vi "(TestVI)RTP Play Test.vi"(5 "RTP Event":refnum<user-event>, 6 "Sampling Rate":u32=8000, 7 "Stop Queue":refnum<queue>, 8 "error in (no error)":errorcluster caption="에러 입력(에러 없음)", 11 "RTP Data":i8[](array[numeric])) -> (0 "error out":errorcluster caption="에러 출력")   [LabVIEW 2020]
uses:
  SubVIs/Serial/Controls/(Ctrl)Serial_Write Read Option.ctl
  f3c870e7-e4f9-4653-aed4-0900bdacb438.vi
  a87611fc-5de5-47b6-9d4c-4620345c1726.vi
  Variables/(Var)System Variables.vi
  SubVIs/Serial/Instance VIs/(SubVI)Serial_Write.vi
  SubVIs/Serial/Instance VIs/(SubVI)Serial_Write-Read.vi
panel:
  out "iteration":i32
  out "Read Array":u8[][](array[numeric])
  out "Current Read":u8[](array[numeric])
  out "time":u32
  out "End Read":u8[](array[numeric])
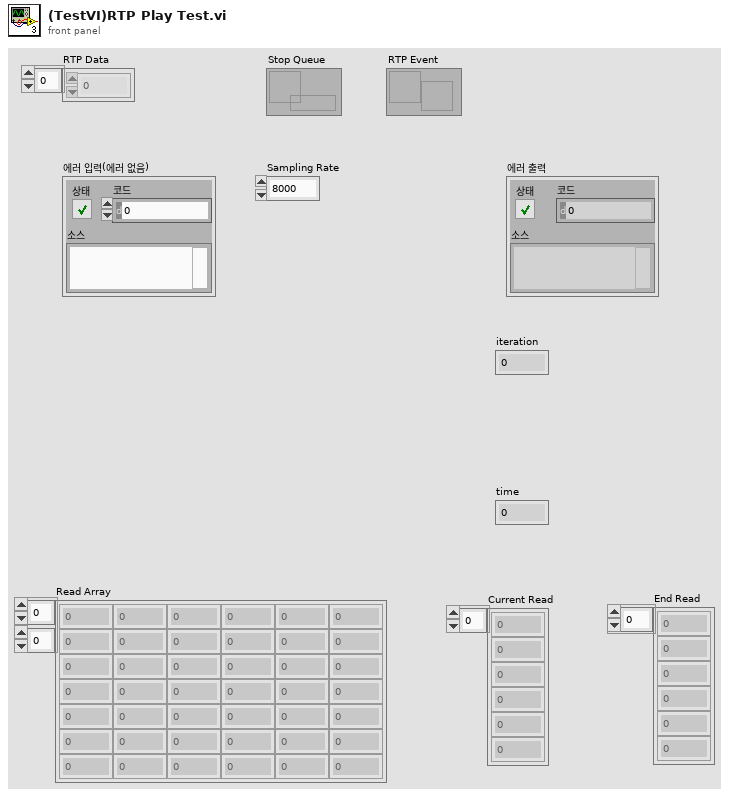
[diagram p1: front panel]
types:
  T1 = typedef "(Ctrl)Serial_Write Read Option.ctl" = cluster{"Echo Request":bool, "Header Verification":bool, "Checksum Verification":bool, "User Code Verifiaction":bool}
  T2 = typedef "Haptic IC.lvclass/(Ctrl)IC Type.ctl" = enum8{"DW7800", "DW7912", "DW7914"}
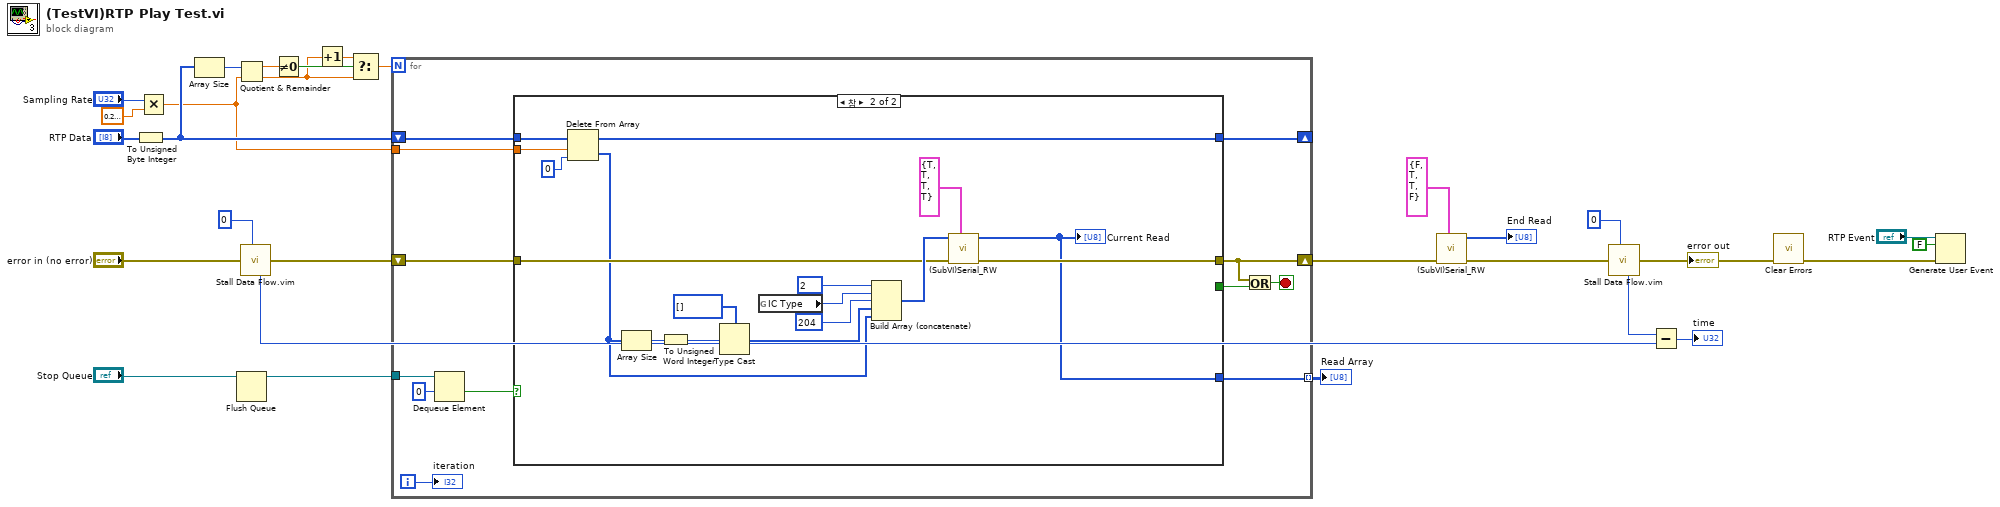
[diagram p0: block diagram]
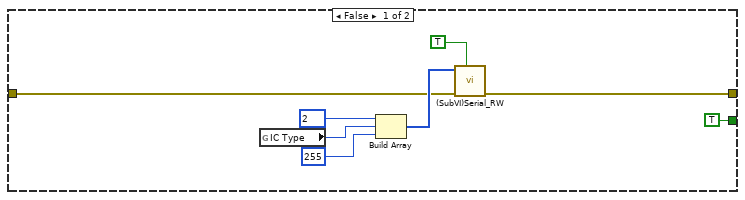
[diagram p2: hidden frame]
diagram:
  n1 = To Unsigned Byte Integer(number="RTP Data") -> (unsigned 8bit integer=w27:u8[])
  n2 = Multiply(x="Sampling Rate", y=0.20000000000000004) -> (x*y=w8:dbl)
  n3 = Array Size(array=w27) -> (size(s)=w26:i32)
  n4 = Flush Queue(queue="Stop Queue") -> (queue out=w6:refnum<queue>)  [unwired: 1 in, 2 out]
  n5 = Quotient & Remainder(x=w26, y=w8) -> (x-y*floor(x/y)=w25:dbl, floor(x/y)=w23:dbl)
  n6 = call "Stall Data Flow.vim"("value in"="error in (no error)", "milliseconds to wait"=u32 0) -> ("millisecond timer value"=w14:u32, "value out"=w18:errorcluster)
  n7 = Not Equal To 0?(x=w25) -> (x != 0?=w24:bool)
  n8 = Increment(x=w23) -> (x+1=w22:dbl)
  n9 = Select(t=w22, s=w24, f=w23) -> (s? t:f=w21:dbl)
  n10 = for {
    N: w21 -> [_]
    shift-right: [w36] -> w19
    shift-left: w18 -> [w41]
    shift-right: [w39] -> _
    shift-left: w27 -> [w40]
    tunnel: [w38] -> w12 mode=indexing
    tunnel: w8 -> [w37]
    tunnel: w6 -> [w32]
    i -> [w35]
    stop <- w34 stop-if-true
    n11 = Dequeue Element(queue=w32, timeout in ms (-1)=0 ("타임아웃(ms) (-1)")) -> (timed out?=w30:bool)  [unwired: 1 in, 3 out]
    n12 = case shown="참" w30 {
      tunnel: w41 -> [w44 w58]
      tunnel: w40 -> [_ w57]
      tunnel: [_ w54] -> w39
      tunnel: [_ w50] -> w38
      tunnel: w37 -> [_ w53]
      tunnel: [w43 w51] -> w36
      tunnel: [TRUE _] -> w33
      frame False {
        n13 = global read "(Var)System Variables.vi" "IC Type"() -> (w47:T2)
        n14 = Build Array(u8 2, w47, u8 255) -> (w48:u8[])
        n15 = call-poly "(SubVI)Serial_RW.vi"("Echo Request"=TRUE, "error in (no error)"=w44, "Data to Write"=w48) -> ("error out"=w43:errorcluster)  [unwired: 8 in]
      }
      frame True {
        n16 = Delete From Array(array=w57, length=w53, index=0 ("인덱스")) -> (deleted portion=w55:u8[], array with subset deleted=w54:u8[])
        n17 = Array Size(array=w55) -> (size(s)=w65:i32)
        n18 = To Unsigned Word Integer(number=w65) -> (unsigned 16bit integer=w64:u16)
        n19 = Type Cast(type=u8[] [] ("타입"), x=w64) -> (*(type *) &x=w62:u8[])
        n20 = global read "(Var)System Variables.vi" "IC Type"() -> (w59:T2)
        n21 = Build Array (concatenate)(u8 2, w59, u8 204, w62, w55) -> (w63:u8[])
        n22 = call-poly "(SubVI)Serial_RW.vi"("Option"=T1 {"Echo Request"=TRUE, "Header Verification"=TRUE, "Checksum Verification"=TRUE, "User Code Verifiaction"=TRUE}, "error in (no error)"=w58, "Data to Write"=w63) -> ("error out"=w51:errorcluster, "Read Data"=w50:u8[])  [unwired: 6 in, 1 out]
        "Current Read" <- w50
      }
    }
    n23 = Or(x=w36, y=w33) -> (x .or. y?=w34:bool)
    "iteration" <- w35
  }
  "Read Array" <- w12
  n24 = call-poly "(SubVI)Serial_RW.vi"("Option"=T1 {"Echo Request"=FALSE, "Header Verification"=TRUE, "Checksum Verification"=TRUE, "User Code Verifiaction"=FALSE}, "error in (no error)"=w19) -> ("error out"=w20:errorcluster, "Read Data"=→"End Read":u8[])  [unwired: 7 in, 1 out]
  n25 = call "Stall Data Flow.vim"("value in"=w20, "milliseconds to wait"=u32 0) -> ("millisecond timer value"=w15:u32, "value out"=w5:errorcluster)
  "error out" <- w5
  n26 = Subtract(x=w15, y=w14) -> (x-y=→"time":u32)
  n27 = call <vilib>:"Clear Errors.vi"("error in (no error)"=w5) -> ("error out"=w2:errorcluster)  [unwired: 5 in, 1 out]
  n28 = Generate User Event(user event="RTP Event", event data cluster=FALSE ("이벤트 데이터"), error in=w2) -> ()  [unwired: 1 in, 2 out]
